vi "Get RT Label Settings for Message.vi"(6 "valid":bool=TRUE, 9 "message identifiers":T11, 10 "map":T2, 11 "RT hardware channel data":T12[](array[typedef]) {"labels settings for RT"."Label Timestamp Channel Data Reference" format="%.0x"; "labels settings for RT"."Word Initial Raw Value" format="%032.0f"; "labels settings for RT"."Label Disable/Trigger Channel Reference" format="%.0x"; "labels settings for RT"."parameter driver data"."Tx parameter refs" format="%.0x"; "labels settings for RT"."SDI" format="%02b"; "labels settings for RT"."label" format="%.0o"}) -> (1 "message indexes":T1, 2 "valid and map exists":bool, 3 "label settings for RT":T3 {"Label Timestamp Channel Data Reference" format="%.0x"; "Word Initial Raw Value" format="%032.0f"; "Label Disable/Trigger Channel Reference" format="%.0x"; "parameter driver data"."Tx parameter refs" format="%.0x"; "SDI" format="%02b"; "label" format="%.0o"})   [LabVIEW 2020, in "AIM ARINC 429 Engine.lvlib" / "Custom Device.lvlib"]
uses:
  Custom Device.lvlib
  Shared/RT Hardware Channel Settings.ctl
  Shared/RT Label Settings.ctl
  Shared/Label.ctl
  Shared/RT Parameters.ctl
  Shared/Parameter Definition.ctl
  <vilib>/NI/NI VeriStand Encoding and Decoding/Encoding.ctl
  <vilib>/NI VeriStand/Custom Device API/Custom Device Item Ref.ctl
  Shared/Transfer Type.ctl
  <vilib>/NI VeriStand/Custom Device API/Data Reference.ctl
  Shared/Map of Identifiers to Indexes.ctl
  <vilib>/NI/NI VeriStand Encoding and Decoding/Encoding and Decoding.lvlib
  <vilib>/NI VeriStand/Custom Device API/Custom Device API.lvlib
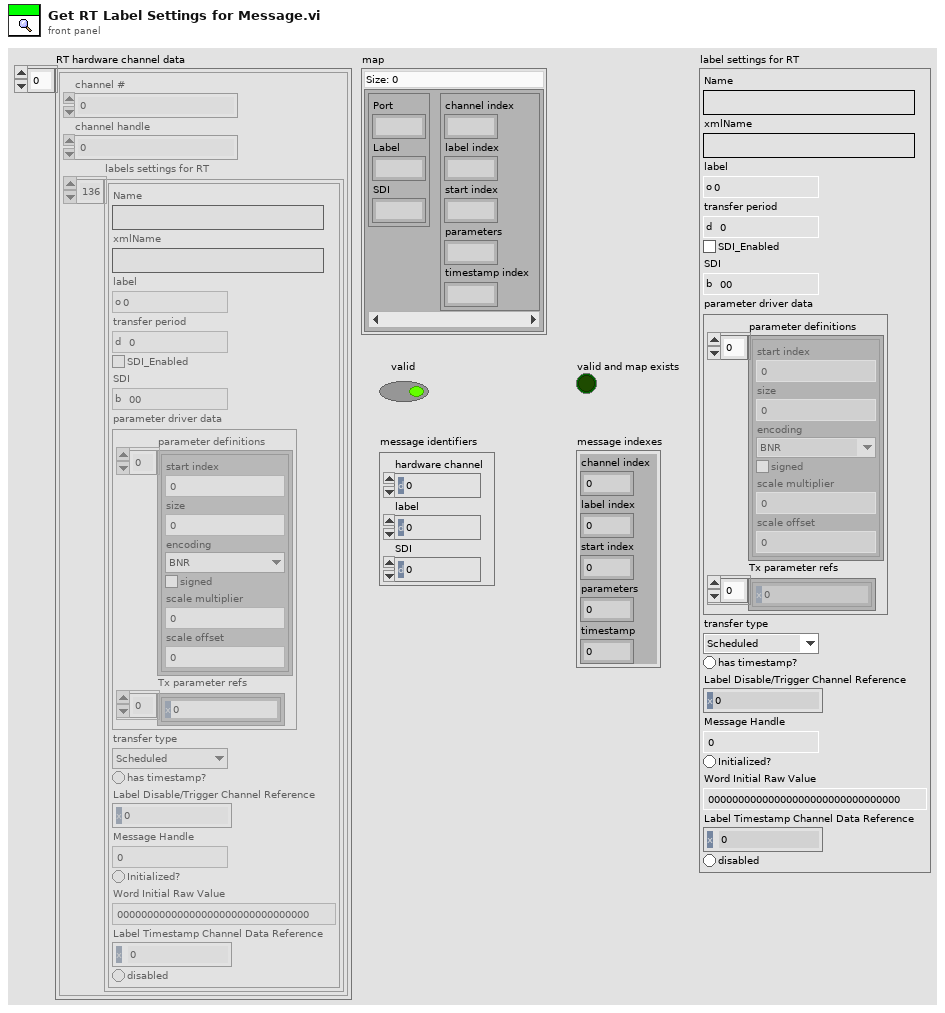
[diagram p1: front panel]
types:
  T1 = cluster{"channel index":i32, "label index":i32, "start index":i32, "parameters":i32, "timestamp":i32}
  T2 = typedef "Map of Identifiers to Indexes.ctl" = map{cluster{"Port":u8, "Label":u8, "SDI":u8}, cluster{"channel index":i32, "label index":i32, "start index":i32, "parameters":i32, "timestamp index":i32}}
  T3 = typedef "RT Label Settings.ctl" = cluster{"Name":string, "xmlName":string, "label":T4, "transfer period":u32, "SDI_Enabled":bool, "SDI":u8, "parameter driver data":T5, "transfer type":T9, "has timestamp?":bool, "Label Disable/Trigger Channel Reference":T8, "Message Handle":u64, "Initialized?":bool, "Word Initial Raw Value":u32, "Label Timestamp Channel Data Reference":T10, "disabled":bool}
  T4 = typedef "Label.ctl" = u8
  T5 = typedef "RT Parameters.ctl" = cluster{"parameter definitions":T6[], "Tx parameter refs":T8[]}
  T6 = typedef "Parameter Definition.ctl" = cluster{"start index":i32, "size":i32, "encoding":T7, "signed":bool, "scale multiplier":dbl, "scale offset":dbl}
  T7 = typedef "Encoding and Decoding.lvlib/Encoding.ctl" = enum16{"BNR", "BCD", "Discrete"}
  T8 = typedef "Custom Device API.lvlib/Custom Device Item Ref.ctl" = u64
  T9 = typedef "Transfer Type.ctl" = enum16{"Scheduled", "Acyclic", "Block", "Strobe"}
  T10 = typedef "Custom Device API.lvlib/Data Reference.ctl" = i32
  T11 = cluster{"hardware channel":u8, "label":u8, "SDI":u8}
  T12 = typedef "RT Hardware Channel Settings.ctl" = cluster{"channel #":u16, "channel handle":u64, "labels settings for RT":T3[]}
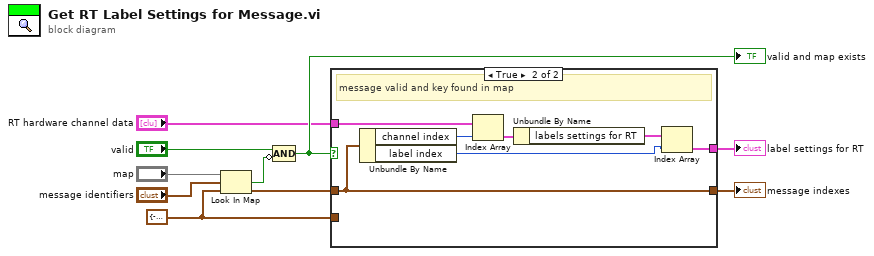
[diagram p0: block diagram]
diagram:
  w1 = T1 {"channel index"=-1, "label index"=-1, "start index"=-1, "parameters"=-1, "timestamp"=-1} ("message info")
  n1 = Look In Map(map="map", key="message identifiers", default value=w1) -> (key not found?=w8:bool, value=w5:T1)
  n2 = Compound Arithmetic op=AND("valid", invert w8) -> (w6:bool)
  "valid and map exists" <- w6
  n3 = case shown="True" w6 {
    tunnel: w5 -> [_ w13]
    tunnel: "RT hardware channel data" -> [_ w18]
    tunnel: [w11 w13] -> w3
    tunnel: [_ w12] -> w2
    tunnel: w1 -> [w11 _]
    frame False {
      # "not valid or not found"
    }
    frame True {
      # "message valid and key found in map"
      n4 = Unbundle By Name(w13) -> ("channel index"=w17:i32, "label index"=w14:i32)
      n5 = Index Array(array=w18, index=w17) -> (element=w16:T12)
      n6 = Unbundle By Name(w16) -> ("labels settings for RT"=w15:T3[])
      n7 = Index Array(array=w15, index=w14) -> (element=w12:T3)
    }
  }
  "label settings for RT" <- w2
  "message indexes" <- w3
